vi "DIM_Read SysLabels (Sourcer).vi"(8 "error in (no error)":errorcluster, 10 "Sourcer":string, 11 "UI_Actor in":refnum<class "UI_Actor.lvclass">) -> (0 "error out":errorcluster, 2 "DIM Sourcer's SysLabels":string[](array[string]), 3 "UI_Actor out":refnum<class "UI_Actor.lvclass">)   [LabVIEW 2020, in "UI_Actor.lvlib" / "UI_Actor.lvclass"]
uses:
  UI_Actor.lvclass
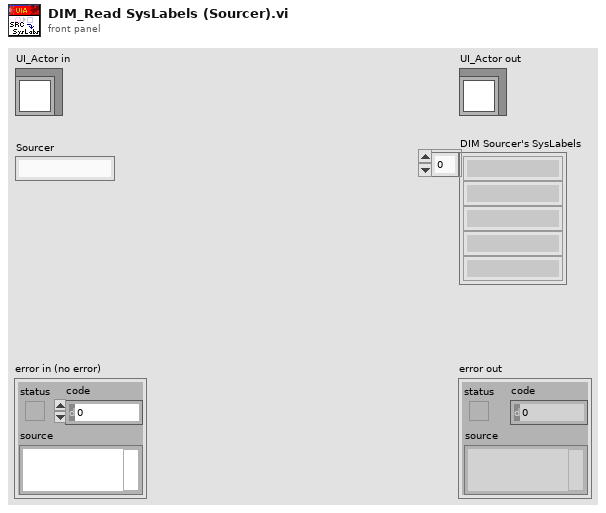
[diagram p1: front panel]
types:
  T1 = typedef "UI_Actor.lvlib/UI_Actor.lvclass/ctl_InternalMapItem.ctl" = cluster{"Config":refnum<class "Config.lvclass">, "LatestData":refnum<class "Data.lvclass">}
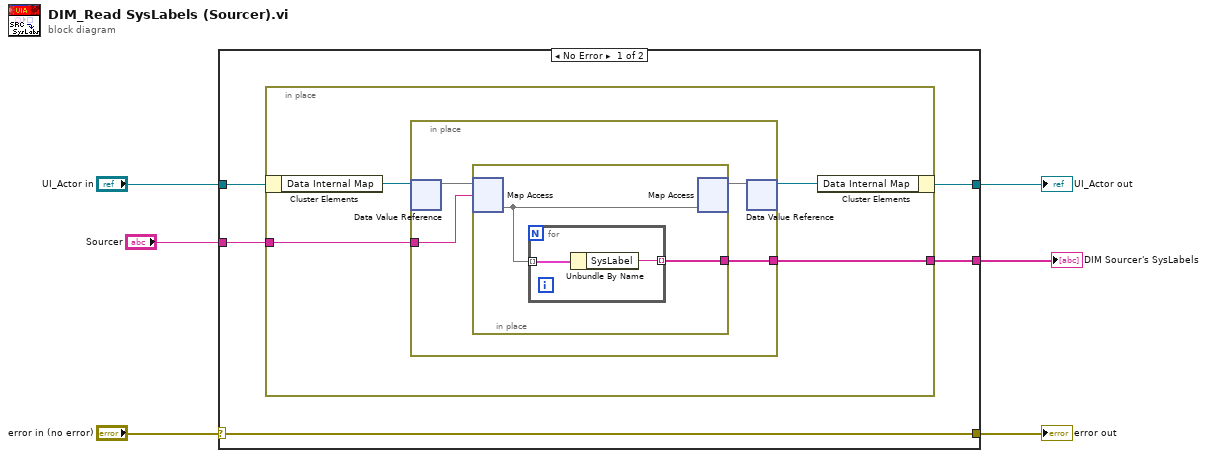
[diagram p0: block diagram]
diagram:
  n1 = case shown="No Error" "error in (no error)" {
    selector: "error in (no error)" -> [w11 w25]
    tunnel: [w11 w25] -> w5
    tunnel: [w9 w24] -> w3
    tunnel: "UI_Actor in" -> [w10 w24]
    tunnel: [w8 _] -> w2
    tunnel: "Sourcer" -> [w7 _]
    frame No Error {
      n2 = in-place {
        in-place-border: [w12] -> w8
        in-place-border: w7 -> [w13]
        n3 = in-place-cluster #1(w10) -> ("Data Internal Map"=w15:refnum<data-value>)
        n4 = in-place {
          in-place-border: w13 -> [w19]
          in-place-border: [w18] -> w12
          n5 = in-place-dvr #2(w15) -> (w17:map{string, map{string, T1}})  [unwired: 1 out]
          n6 = in-place {
            in-place-border: [w21] -> w18
            n7 = in-place-map #3(w17, w19) -> (w20:map{string, T1})  [unwired: 1 in, 1 out]
            n8 = for {
              tunnel: w20 -> [w23] mode=indexing
              tunnel: [w22] -> w21 mode=indexing
              n9 = Unbundle By Name(w23) -> ("SysLabel"=w22:string)
            }
            n10 = in-place-map #3(w20) -> (w16:map{string, map{string, T1}})  [unwired: 1 in, 2 out]
          }
          n11 = in-place-dvr #2(w16) -> (w14:refnum<data-value>)  [unwired: 1 out]
        }
        n12 = in-place-cluster #1("Data Internal Map"=w14) -> (w9:refnum<class "UI_Actor.lvclass">)
      }
    }
    frame Error {
    }
  }
  "error out" <- w5
  "UI_Actor out" <- w3
  "DIM Sourcer's SysLabels" <- w2
